vi "Write.vi"(8 "error in (no error)":errorcluster, 9 "timeout (2000 ms)":i32=2000, 10 "Bytes":u8[](array[numeric]) format="%08b", 11 "Connection in":refnum<class "Connection.lvclass">) -> (0 "error out":errorcluster, 3 "Connection":refnum<class "Connection.lvclass">)   [LabVIEW 2013, in "Connection_GOSPL.lvlib" / "Connection.lvclass"]
uses:
  Connection.lvclass
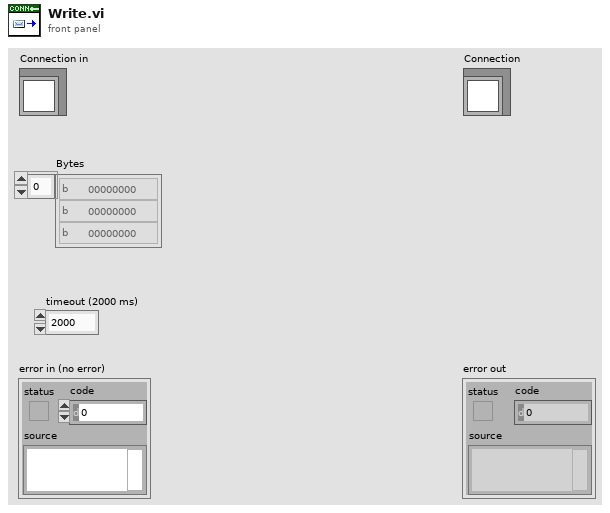
[diagram p1: front panel]
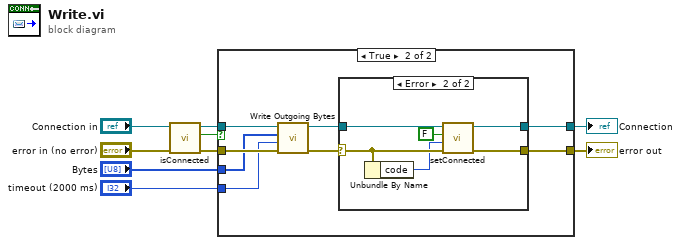
[diagram p0: block diagram]
diagram:
  n1 = call "isConnected.vi"("error in (no error)"="error in (no error)", "Connection in"="Connection in") -> ("error out"=w8:errorcluster, "connected"=w7:bool, "Connection out"=w9:refnum<class "Connection.lvclass">)  [unwired: 7 in]
  n2 = case shown="True" w7 {
    tunnel: "Bytes" -> [_ w15]
    tunnel: "timeout (2000 ms)" -> [_ w14]
    tunnel: [w11 w13] -> w4
    tunnel: [w10 w12] -> w3
    tunnel: w9 -> [w11 w19]
    tunnel: w8 -> [w10 w18]
    frame False {
    }
    frame True {
      n3 = call-dynamic "Write Outgoing Bytes.vi"("error in (no error)"=w18, "timeout (2000 ms)"=w14, "Bytes"=w15, "Connection in"=w19) -> ("error out"=w17:errorcluster, "Connection out"=w16:refnum<class "Connection.lvclass">)  [unwired: 6 in]
      n4 = case shown="Error" w17 {
        selector: w17 -> [w20 w24]
        tunnel: [w20 w25] -> w12
        tunnel: w16 -> [w21 w27]
        tunnel: [w21 w26] -> w13
        frame No Error {
        }
        frame Error {
          n5 = Unbundle By Name(w24) -> ("code"=w23:i32)
          n6 = call "setConnected.vi"("error in (no error)"=w24, "reason"=w23, "connected"=FALSE, "Connection in"=w27) -> ("error out"=w25:errorcluster, "Connection out"=w26:refnum<class "Connection.lvclass">)  [unwired: 6 in]
        }
      }
    }
  }
  "error out" <- w3
  "Connection" <- w4
